vi "ICM Read MICAS-X Channel List.vi"() -> (2 "Channels":string[](array[string]), 3 "Import?":bool)   [LabVIEW 2024]
doc: "ICM Read MICAS-X Channel List.vi\n\nThis VI is used by the General Parser Editor to read a Channel List from a MICAS-X configuration file and set up the parsing to work with that list.\n\nInstrument Communication Module Version 1.0\nJune 2025 Original Code Consulting David Thomson\n www.originalcode.com"
panel:
  in  "Cancel":bool
  in  "Import":bool
  in  "Lists":u16(ring)
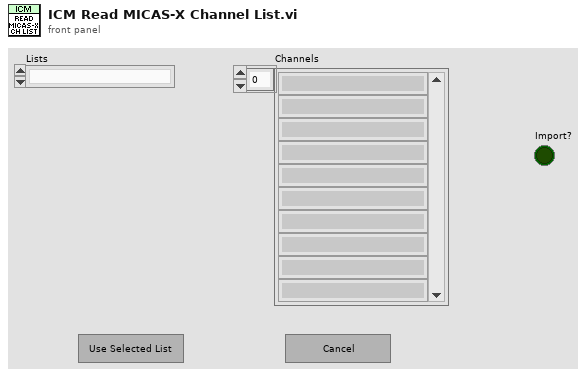
[diagram p1: front panel]
types:
  T1 = enum8{"Enabled", "Disabled", "Disabled and Grayed Out"}
  T2 = cluster{"Lists":cluster{"List Name":string, "Channels":string[]}[], "Notes":string}
  T3 = cluster{"List Name":string, "Channels":string[]}[]
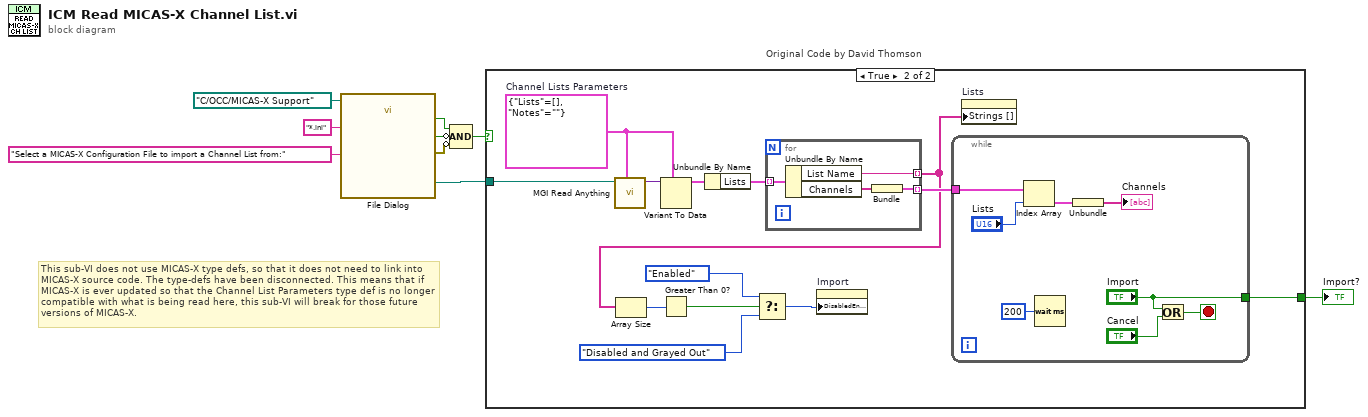
[diagram p0: block diagram]
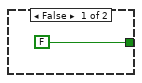
[diagram p2: hidden frame]
diagram:
  # "This sub-VI does not use MICAS-X type defs, so that it does not need to link into\nMICAS-X source code. The type-defs have been disconnected. This means that if\nMICAS-X is ever updated so that the Channel List Parameters type def is no longer\ncompatible with what is being read here, this sub-VI will break for those future\nversions of MICAS-X."
  n1 = call "File Dialog"("start path"=path "C:/OCC/MICAS-X Support", "prompt"="Select a MICAS-X Configuration File to import a Channel List from:", "pattern (all files)"="*.ini") -> ("selected path"=w2:path, "exists"=w6:bool, "cancelled"=w5:bool, "error out"=w4:errorcluster)  [unwired: 9 in]
  n2 = Compound Arithmetic op=AND(w6, invert w5, invert w4) -> (w3:bool)
  n3 = case "Original Code by David Thomson" shown="True" w3 {
    tunnel: w2 -> [_ w23]
    tunnel: [FALSE ("Import") w18] -> w1
    frame False {
    }
    frame True {
      w22 = T2 {"Lists"=[], "Notes"=""}  # Channel Lists Parameters
      n4 = call <userlib>:"MGI Read Anything.vi"("Type of Anything"=w22, "Path (dialog)"=w23) -> ("Anything"=w21:variant)  [unwired: 6 in, 3 out]
      n5 = Variant To Data(type=w22, Variant=w21) -> (data=w20:T2)  [unwired: 1 in, 1 out]
      n6 = Unbundle By Name(w20) -> ("Lists"=w19:T3)
      n7 = for {
        tunnel: w19 -> [w35] mode=indexing
        tunnel: [w34] -> w16 mode=indexing
        tunnel: [w32] -> w17 mode=indexing
        n8 = Unbundle By Name(w35) -> ("List Name"=w34:string, "Channels"=w33:string[])
        n9 = Bundle("Channels"=w33) -> (w32:cluster{"Channels":string[]})  [unwired: 1 in]
      }
      n10 = Array Size(array=w16) -> (size(s)=w15:i32)
      n11 = Greater Than 0?(x=w15) -> (x > 0?=w14:bool)
      n12 = Select(t=T1."Enabled" ("Disabled"), s=w14, f=T1."Disabled and Grayed Out" ("Disabled")) -> (s? t:f=w12:T1)
      n13 = property on="Import" class="Bool"("DisabledEnum"=w12) -> ()  [unwired: 2 in, 2 out]
      n14 = while {
        tunnel: ["Import"] -> w18
        tunnel: w17 -> [w26]
        stop <- w29 stop-if-true
        n15 = Index Array(array=w26, index="Lists") -> (element=w25:cluster{"Channels":string[]})
        n16 = Wait (ms)(milliseconds to wait=u32 200) -> ()  [unwired: 1 out]
        n17 = Unbundle(w25) -> ("Channels"=→"Channels":string[])
        n18 = Or(x="Import", y="Cancel") -> (x .or. y?=w29:bool)
      }
      n19 = property on="Lists" class="Ring (strict)"("Strings []"=w16) -> ()  [unwired: 2 in, 2 out]
    }
  }
  "Import?" <- w1
